vi "Write PF Commands Msg.vi"(10 "Platform.lvlib:PF Commands Msg.lvclass":refnum<class "PF Commands Msg.lvclass">, 11 "Platform in":refnum<class "Platform.lvclass">) -> (3 "Platform out":refnum<class "Platform.lvclass">)   [LabVIEW 2019, in "Platform.lvlib" / "Platform.lvclass"]
uses:
  Platform.lvclass
  Platform Messages/Run Msg/PF Commands Msg.lvclass
  Platform.lvclass/Platform.ctl
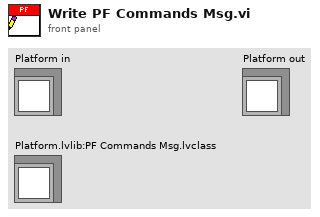
[diagram p1: front panel]
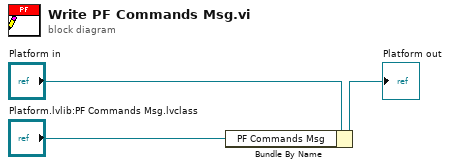
[diagram p0: block diagram]
diagram:
  n1 = Bundle By Name(cluster="Platform in", "PF Commands Msg"="Platform.lvlib:PF Commands Msg.lvclass") -> (→"Platform out":refnum<class "Platform.lvclass">)
